vi "Stop.vi"(8 "error in":errorcluster, 11 "Scope Base in":refnum<class "Scope Base.lvclass">) -> (0 "error out":errorcluster, 3 "Scope Base out":refnum<class "Scope Base.lvclass">)   [LabVIEW 2023, in "Scope.lvlib" / "Scope Base.lvlib" / "Scope Base.lvclass"]
uses:
  Scope Base.lvclass
  Scope Base.lvclass/Scope Base.ctl
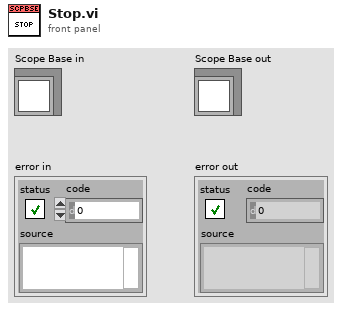
[diagram p1: front panel]
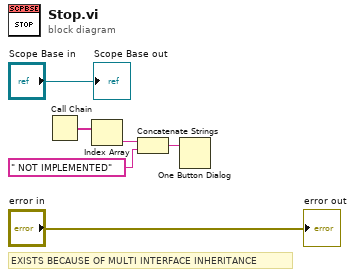
[diagram p0: block diagram]
diagram:
  # "EXISTS BECAUSE OF MULTI INTERFACE INHERITANCE"
  n1 = Call Chain() -> (call chain=w6:string[])
  n2 = Index Array(array=w6) -> (element=w4:string)  [unwired: 1 in]
  n3 = Concatenate Strings(w4, " NOT IMPLEMENTED" ("string")) -> (w5:string)
  n4 = One Button Dialog(message=w5) -> ()  [unwired: 1 in, 1 out]
  "error out" <- "error in"
  "Scope Base out" <- "Scope Base in"
